vi "ConfigureHyperscope.vi"() -> ()   [LabVIEW 2012]
uses:
  <vilib>/Utility/config.llb/Write Key (String).vi
  <vilib>/Utility/config.llb/NI_LVConfig.lvlib
panel:
  in  "Cancel":bool
  in  "Confirm":bool
  in  "Switch (Linkbone) Serial Port":refnum<visa-resource-name>
  in  "DAQ Package":enum16{"RGG_GG", "RG_GG", "GG_GG", "RGG"}(ring)
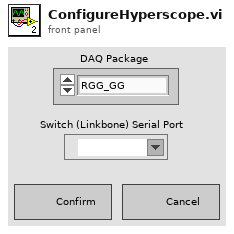
[diagram p1: front panel]
types:
  T1 = typedef "NI_LVConfig.lvlib/Config Data RefNum.ctl" = refnum<k1>
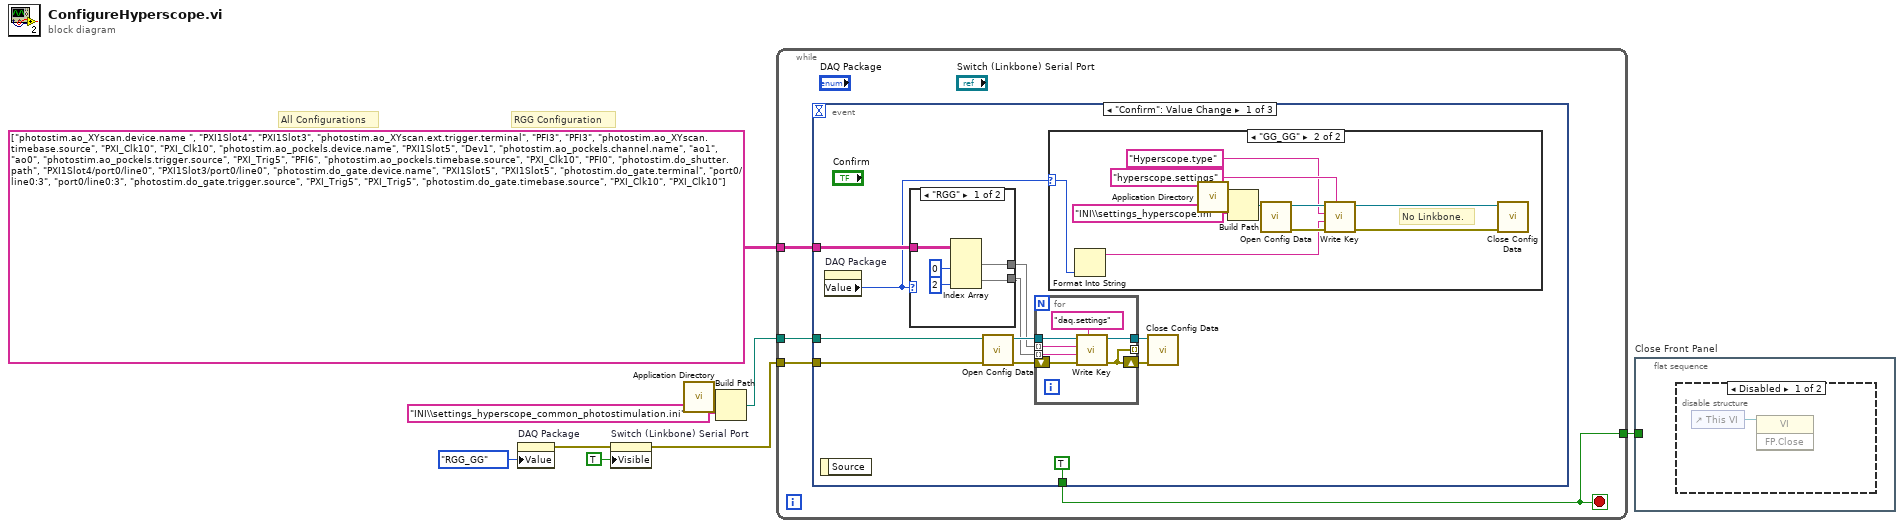
[diagram p0: block diagram]
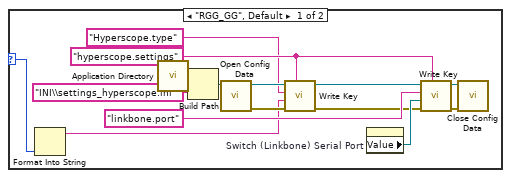
[diagram p3: hidden frame]
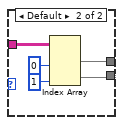
[diagram p4: hidden frame]
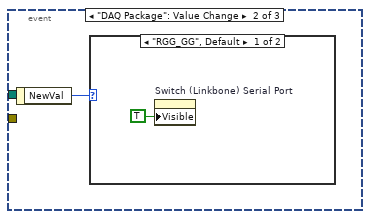
[diagram p5: hidden frame]
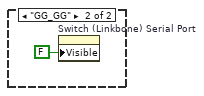
[diagram p6: hidden frame]
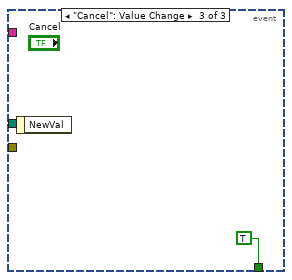
[diagram p7: hidden frame]
diagram:
  # "RGG Configuration"
  # "All Configurations"
  n1 = property on="DAQ Package" class="Enum (strict)"("Value"=enum16{"RGG_GG", "RG_GG", "GG_GG", "RGG"}."RGG_GG" ("DAQ Package")) -> (error out=w4:errorcluster)  [unwired: 2 in, 1 out]
  n2 = property on="Switch (Linkbone) Serial Port" class="VISAName"(error in=w4, "Visible"=TRUE) -> (error out=w1:errorcluster)  [unwired: 1 in, 1 out]
  n3 = call <vilib>:"Application Directory.vi"() -> ("Application Directory"=w8:path)
  n4 = Build Path(base path=w8, name or relative path="INI\\settings_hyperscope_common_photostimulation.ini") -> (appended path=w2:path)
  n5 = while {
    tunnel: [w13] -> w9
    tunnel: string[][] [["photostim.ao_XYscan.device.name ", "PXI1Slot4", "PXI1Slot3"], ["photostim.ao_XYscan.ext.trigger.terminal", "PFI3", "PFI3"], ["photostim.ao_XYscan.timebase.source", "PXI_Clk10", "PXI_Clk10"], ["photostim.ao_pockels.device.name", "PXI1Slot5", "Dev1"], ["photostim.ao_pockels.channel.name", "ao1", "ao0"], ["photostim.ao_pockels.trigger.source", "PXI_Trig5", "PFI6"], ["photostim.ao_pockels.timebase.source", "PXI_Clk10", "PFI0"], ["photostim.do_shutter.path", "PXI1Slot4/port0/line0", "PXI1Slot3/port0/line0"], ["photostim.do_gate.device.name", "PXI1Slot5", "PXI1Slot5"], ["photostim.do_gate.terminal", "port0/line0:3", "port0/line0:3"], ["photostim.do_gate.trigger.source", "PXI_Trig5", "PXI_Trig5"], ["photostim.do_gate.timebase.source", "PXI_Clk10", "PXI_Clk10"]] -> [w12]
    tunnel: w2 -> [w11]
    tunnel: w1 -> [w10]
    stop <- w13 stop-if-true
    n6 = event shown="[0] \"Confirm\": Value Change" {
      selector: _ -> [_ _ _]
      dyn-events: _ -> [_ _ _]
      timeout: _ -> [_ _ _]
      tunnel: [TRUE _ TRUE] -> w13
      tunnel: w12 -> [w23 _ _]
      tunnel: w11 -> [w22 _ _]
      tunnel: w10 -> [w21 _ _]
      event "Confirm": Value Change {
        n7 = event-data() -> ()  [unwired: 1 in, 1 out]
        n8 = property on="DAQ Package" class="Enum (strict)"() -> ("Value"=w14:enum16{"RGG_GG", "RG_GG", "GG_GG", "RGG"})  [unwired: 2 in, 2 out]
        n9 = case shown="\"RGG\"" w14 {
          tunnel: w23 -> [w62 w67]
          tunnel: [w59 w64] -> w17
          tunnel: [w58 w63] -> w18
          frame "RGG" {
            n10 = Index Array(array=w62, index (col) #1=0 ("disabled index (col)"), index (col) #2=2 ("index (col)")) -> (element #1=w58:string[], element #2=w59:string[])  [unwired: 2 in]
          }
          frame Default {
            n11 = Index Array(array=w67, index (col) #1=0 ("disabled index (col)"), index (col) #2=1 ("index (col)")) -> (element #1=w63:string[], element #2=w64:string[])  [unwired: 2 in]
          }
        }
        n12 = call <vilib>:"Open Config Data.vi"("error in (no error)"=w21, "configuration file path"=w22) -> ("error out"=w19:errorcluster, "refnum"=w20:T1)  [unwired: 7 in, 1 out]
        n13 = for {
          tunnel: w20 -> [w56]
          tunnel: w18 -> [w54] mode=indexing
          tunnel: w17 -> [w51] mode=indexing
          shift-right: [w52] -> w15
          shift-left: w19 -> [w55]
          tunnel: [w53] -> w16
          tunnel: [w52] -> _ mode=indexing
          n14 = call-poly <vilib>:"Write Key.vi"("section"="daq.settings", "error in (no error)"=w55, "value"=w51, "key"=w54, "refnum"=w56) -> ("error out"=w52:errorcluster, "refnum out"=w53:T1)  [unwired: 4 in, 1 out]
        }
        n15 = case shown="\"GG_GG\"" w14 {
          selector: w14 -> [w26 w43]
          frame "RGG_GG", Default {
            w29 = "hyperscope.settings" ("section")
            n16 = Format Into String(w26) -> (resulting string=w25:string)  [unwired: 3 in, 1 out]
            n17 = call <vilib>:"Application Directory.vi"() -> ("Application Directory"=w35:path)
            n18 = Build Path(base path=w35, name or relative path="INI\\settings_hyperscope.ini") -> (appended path=w36:path)
            n19 = call <vilib>:"Open Config Data.vi"("configuration file path"=w36) -> ("error out"=w32:errorcluster, "refnum"=w33:T1)  [unwired: 8 in, 1 out]
            n20 = call-poly <vilib>:"Write Key.vi"("section"=w29, "error in (no error)"=w32, "value"=w25, "key"="Hyperscope.type", "refnum"=w33) -> ("error out"=w30:errorcluster, "refnum out"=w31:T1)  [unwired: 4 in, 1 out]
            n21 = property on="Switch (Linkbone) Serial Port" class="VISAName"() -> ("Value"=w34:refnum<visa-resource-name>)  [unwired: 2 in, 2 out]
            n22 = call-poly <vilib>:"Write Key.vi"("section"=w29, "error in (no error)"=w30, "value"=w34, "key"="linkbone.port", "refnum"=w31) -> ("error out"=w39:errorcluster, "refnum out"=w38:T1)  [unwired: 4 in, 1 out]
            n23 = call <vilib>:"Close Config Data.vi"("error in (no error)"=w39, "refnum"=w38) -> ()  [unwired: 8 in, 2 out]
          }
          frame "GG_GG" {
            # "No Linkbone."
            n24 = Format Into String(w43) -> (resulting string=w42:string)  [unwired: 3 in, 1 out]
            n25 = call <vilib>:"Application Directory.vi"() -> ("Application Directory"=w49:path)
            n26 = Build Path(base path=w49, name or relative path="INI\\settings_hyperscope.ini") -> (appended path=w50:path)
            n27 = call <vilib>:"Open Config Data.vi"("configuration file path"=w50) -> ("error out"=w47:errorcluster, "refnum"=w48:T1)  [unwired: 8 in, 1 out]
            n28 = call-poly <vilib>:"Write Key.vi"("section"="hyperscope.settings", "error in (no error)"=w47, "value"=w42, "key"="Hyperscope.type", "refnum"=w48) -> ("error out"=w40:errorcluster, "refnum out"=w41:T1)  [unwired: 4 in, 1 out]
            n29 = call <vilib>:"Close Config Data.vi"("error in (no error)"=w40, "refnum"=w41) -> ()  [unwired: 8 in, 2 out]
          }
        }
        n30 = call <vilib>:"Close Config Data.vi"("error in (no error)"=w15, "refnum"=w16) -> ()  [unwired: 8 in, 2 out]
      }
      event "DAQ Package": Value Change {
        n31 = event-data() -> ("NewVal"=w68:enum16{"RGG_GG", "RG_GG", "GG_GG", "RGG"})  [unwired: 1 in]
        n32 = case shown="\"RGG_GG\", Default" w68 {
          frame "RGG_GG", Default {
            n33 = property on="Switch (Linkbone) Serial Port" class="VISAName"("Visible"=TRUE) -> ()  [unwired: 2 in, 2 out]
          }
          frame "GG_GG" {
            n34 = property on="Switch (Linkbone) Serial Port" class="VISAName"("Visible"=FALSE) -> ()  [unwired: 2 in, 2 out]
          }
        }
      }
      event "Cancel": Value Change {
        n35 = event-data() -> ()  [unwired: 1 in, 1 out]
      }
    }
  }
  n36 = flat-sequence "Close Front Panel" {
    tunnel: w9 -> [_]
    frame #0 {
      n37 = disable-structure shown="Disabled" {
        frame Disabled {
          n38 = control-ref of="This VI"() -> (w72:refnum<vi>)
          n39 = invoke class="VI" method="FP.Close"(reference=w72) -> ()  [unwired: 2 in, 3 out]
        }
        frame Enabled {
        }
      }
    }
  }
